vi "Test Control Drag.vi"(0 "FSM.Edge In":refnum<class "FSM.Edge.lvclass">, 9 "Coords":T1) -> (4 "FSM.Edge Out":refnum<class "FSM.Edge.lvclass">, 8 "drag control?":bool, 10 "attached node":string)   [LabVIEW 2020, in "FSM.Edge.lvclass"]
uses:
  FSM.Edge.lvclass
  <vilib>/Utility/miscctls.llb/LVPoint32TypeDef.ctl
  FSM.Edge.lvclass/FSM.Edge.ctl
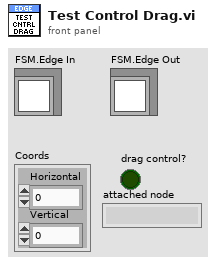
[diagram p1: front panel]
types:
  T1 = typedef "LVPoint32TypeDef.ctl" = cluster{"Horizontal":i32, "Vertical":i32}
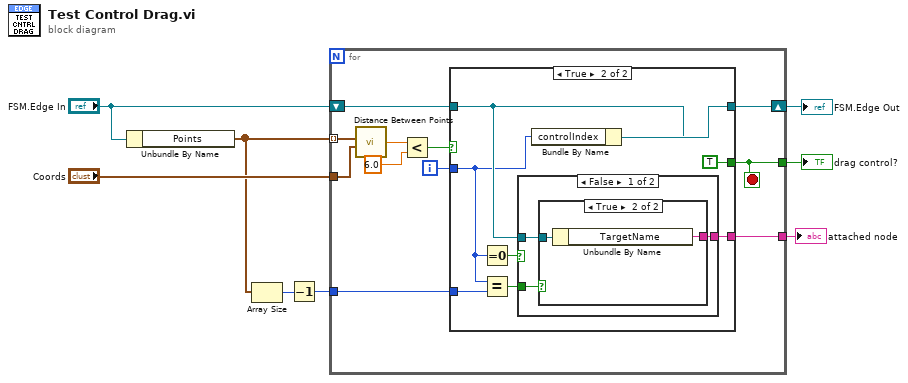
[diagram p0: block diagram]
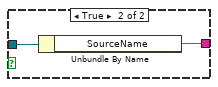
[diagram p4: hidden frame]
diagram:
  n1 = Unbundle By Name("FSM.Edge In") -> ("Points"=w3:cluster{"x":i16, "y":i16}[])
  n2 = Array Size(array=w3) -> (size(s)=w4:i32)
  n3 = Decrement(x=w4) -> (x-1=w2:i32)
  n4 = for {
    shift-right: [w18] -> w7
    shift-left: "FSM.Edge In" -> [w19]
    tunnel: w3 -> [w17] mode=indexing
    tunnel: "Coords" -> [w16]
    tunnel: [w12] -> w5
    tunnel: [w10] -> w1
    tunnel: w2 -> [w9]
    i -> [w11]
    stop <- w12 stop-if-true
    n5 = call "Distance Between Points.vi"("B"=w16, "A"=w17) -> ("distance"=w15:dbl)  [unwired: 4 in]
    n6 = Less?(x=w15, y=6.0) -> (x < y?=w13:bool)
    n7 = case shown="True" w13 {
      tunnel: w19 -> [w20 w25]
      tunnel: [w20 w28] -> w18
      tunnel: [_ TRUE] -> w12
      tunnel: w11 -> [_ w22]
      tunnel: [_ w24] -> w10
      tunnel: w9 -> [_ w23]
      frame False {
      }
      frame True {
        n8 = Equal To 0?(x=w22) -> (x = 0?=w26:bool)
        n9 = Equal?(x=w22, y=w23) -> (x = y?=w21:bool)
        n10 = case shown="False" w26 {
          tunnel: w25 -> [w31 w35]
          tunnel: [w29 w34] -> w24
          tunnel: w21 -> [w30 _]
          frame False {
            n11 = case shown="True" w30 {
              tunnel: w31 -> [_ w33]
              tunnel: [_ w32] -> w29
              frame False {
              }
              frame True {
                n12 = Unbundle By Name(w33) -> ("TargetName"=w32:string)
              }
            }
          }
          frame True {
            n13 = Unbundle By Name(w35) -> ("SourceName"=w34:string)
          }
        }
        n14 = Bundle By Name(cluster=w25, "controlIndex"=w22) -> (w28:refnum<class "FSM.Edge.lvclass">)
      }
    }
  }
  "FSM.Edge Out" <- w7
  "drag control?" <- w5
  "attached node" <- w1
